vi "FPGA_DIOWriteDO_PWMConfig.vi"(7 "DO_PWMPeriodPower":u16, 8 "error in (no error)":errorcluster, 9 "DO_PWM Index":i8, 10 "DO_PWMOutputSelect":T1=enum."DIO 1", 11 "DIODeviceRef":T2) -> (0 "error out":errorcluster, 2 "DO_PWMPeriodPower Out":u16, 3 "DIODeviceRef":T2)   [LabVIEW 2017]
uses:
  <vilib>/Rock Robotics/SystemInterfaces/DIO/FPGA_DIODevRef.ctl
  <vilib>/Rock Robotics/SystemInterfaces/DIO/FPGA_DIOChannel.ctl
  <vilib>/Rock Robotics/SystemInterfaces/System/FPGA_SystemFPGA Ref Global.vi
  <vilib>/Utility/error.llb/Error Cluster From Error Code.vi
  <vilib>/rvi/errors/niLvFpgaAdjustHostInterfaceError.vi
  <vilib>/rvi/interface/nirviReadWriteControl/nirviReadWriteControl.xnode
  <vilib>/Rock Robotics/SystemInterfaces/System/FPGA_SystemFRC FPGA Ref.ctl
  <vilib>/rvi/interface/Simulation/niFpgaSimulationCallBeginRW.vi
  NiFpgaLv.dll
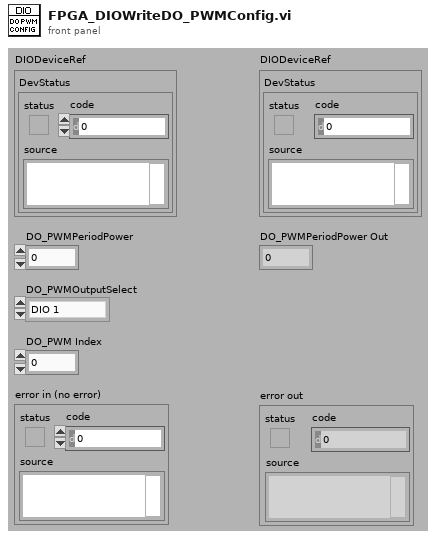
[diagram p1: front panel]
types:
  T1 = typedef "FPGA_DIOChannel.ctl" = enum8{"DIO 0", "DIO 1", "DIO 2", "DIO 3", "DIO 4", "DIO 5", "DIO 6", "DIO 7", "DIO 8", "DIO 9", "DIO MXP 0", "DIO MXP 1", "DIO MXP 2", "DIO MXP 3", "DIO MXP 4", "DIO MXP 5", "DIO MXP 6", "DIO MXP 7", "DIO MXP 8", "DIO MXP 9", "DIO MXP 10", "DIO MXP 11", "DIO MXP 12", "DIO MXP 13", "DIO MXP 14", "DIO MXP 15", "SPI Port CS1", "SPI Port CS2", "SPI Port CS3", "SPI Port MISO", "SPI Port MOSI", "Invalid"}
  T2 = typedef "FPGA_DIODevRef.ctl" = cluster{"DevStatus":errorcluster}
  T3 = typedef "FPGA_SystemFRC FPGA Ref.ctl" = refnum<k20>
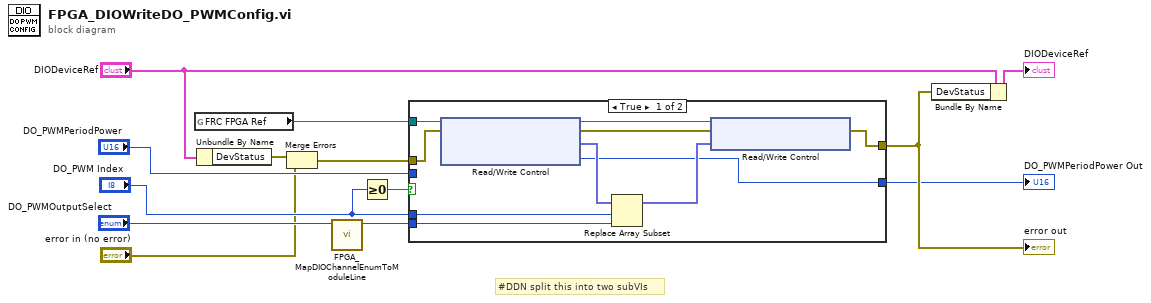
[diagram p0: block diagram]
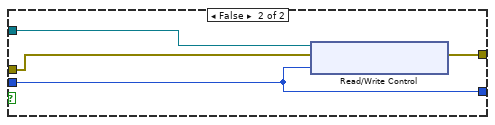
[diagram p2: hidden frame]
diagram:
  # "#DDN split this into two subVIs"
  n1 = global read "FPGA_SystemFPGA Ref Global.vi" "FRC FPGA Ref"() -> (w6:T3)
  n2 = Unbundle By Name("DIODeviceRef") -> ("DevStatus"=w5:errorcluster)
  n3 = Merge Errors(w5, "error in (no error)") -> (w4:errorcluster)
  n4 = call <vilib>:"FPGA_MapDIOChannelEnumToModuleLine.vi"("DIOChannel"="DO_PWMOutputSelect") -> ("ActualDIOChannel(U8)"=w7:u8)  [unwired: 10 out]
  n5 = Greater Or Equal To 0?(x="DO_PWM Index") -> (x >= 0?=w2:bool)
  n6 = case shown="True" w2 {
    tunnel: [w21 w27] -> w12
    tunnel: "DO_PWM Index" -> [w20 _]
    tunnel: w7 -> [w19 _]
    tunnel: [w14 w24] -> w8
    tunnel: w6 -> [w18 w26]
    tunnel: w4 -> [w17 w25]
    tunnel: "DO_PWMPeriodPower" -> [_ w24]
    frame True {
      n7 = xnode "Read/Write Control"("FPGA VI Reference In"=w18, "error in"=w17) -> ("FPGA VI Reference Out"=w22:T3, "error out"=w23:errorcluster, "DIO.PWMOutputSelect"=w16:fxp<+,5,5>[], "DIO.PWMPeriodPower"=w14:u16)
      n8 = Replace Array Subset(array=w16, new element=w19, index=w20) -> (w15:fxp<+,5,5>[])
      n9 = xnode "Read/Write Control"("FPGA VI Reference In"=w22, "error in"=w23, "DIO.PWMOutputSelect"=w15) -> ("error out"=w21:errorcluster)  [unwired: 1 out]
    }
    frame False {
      n10 = xnode "Read/Write Control"("FPGA VI Reference In"=w26, "error in"=w25, "DIO.PWMPeriodPower"=w24) -> ("error out"=w27:errorcluster)  [unwired: 1 out]
    }
  }
  "error out" <- w12
  "DO_PWMPeriodPower Out" <- w8
  n11 = Bundle By Name(cluster="DIODeviceRef", "DevStatus"=w12) -> (→"DIODeviceRef":T2)
